vi "MasterAquisitionFile_FP_Shak.vi"() -> ()   [LabVIEW 2020]
uses:
  <vilib>/vision/driver/IMAQdx.llb/IMAQdx Camera Control Mode.ctl
  <vilib>/vision/driver/IMAQdx.llb/IMAQdx Acquisition Mode.ctl
  <vilib>/userDefined/High Color/IMAQdx.ctl
  <vilib>/vision/driver/IMAQdx.llb/IMAQdx Buffer Number Mode.ctl
  <vilib>/DAQmx/read.llb/DAQmx Read (Analog 1D Wfm NChan NSamp).vi
  <vilib>/DAQmx/create/channels.llb/DAQmx Create Channel (AI-Voltage-Basic).vi
  <vilib>/DAQmx/configure/timing.llb/DAQmx Timing (Sample Clock).vi
  <vilib>/DAQmx/configure/trigger.llb/DAQmx Start Trigger (Digital Edge).vi
  <vilib>/DAQmx/create/channels.llb/DAQmx Create Channel (CO-Pulse Generation-Frequency).vi
  <vilib>/DAQmx/configure/timing.llb/DAQmx Timing (Implicit).vi
  <vilib>/DAQmx/miscellaneous.llb/DAQmx Fill In Error Info.vi
  <vilib>/vision/driver/NI_Vision_Acquisition_Software.lvlib
  <resource>/objmgr/imaqdx.rc
panel:
  in  "Analog Input Channels":tag="Dev1/ai3:5, Dev1/ai8:13"
  out "?":T1(plugin-control)
  in  "stop":bool
  out "?":T1(plugin-control)
  out "Behavior Cam Fs":dbl(knob)=12.024443130297655 scale=0.0..200.0
  out "Behav Cam":bool=TRUE
  out "Whisk Cam":bool=TRUE
  out "Analog Data":bool=TRUE
  out "Time Elapsed (Min)":cluster{dbl, dbl}(slide)={15.0, 10.85073638} scale=0.0..16.0 scale format="%#_2g"
  out "Saving":bool
  out "Analog Samples":i32=13018238
  in  "Device Analog Channel Labels":string[](array[string])=["AudSol", "forceSensor", "560LH", "hipp", "cortRH", "cortLH", "EMG", "LPadSol", "RPadSol"]
  in  "?":cluster{"Analog Fs":u16}={"Analog Fs"=20000} {"Analog Fs" format="%0.0f"}
  in  "?":cluster{"WhiskerCam Fs":u16}={"WhiskerCam Fs"=150}
  out "Notes Size":i32=7
  out "Notes Reversed":string[](array[string])=["Experimenter", "Animal ID", "Isoflurane time", "Amplifier Gain", "Session ID", "Hemisphere", "Solenoid PSI"]
  out "Notes Array":string[](array[string])=["Solenoid PSI", "Hemisphere", "Session ID", "Amplifier Gain", "Isoflurane time", "Animal ID", "Experimenter"]
  in  "Notes:":T2={"Experimenter"="Kevin\n", "Animal ID"="T251", "Isoflurane time"="0940", "Amplifier Gain"="10000", "Session ID"="Imaging Session One", "Hemisphere"="RH", "Solenoid PSI"="10"}
  in  "Target Path":path=path "C:/LabViewData/Bilateral/T251/Imaging Session 1 - 28 Feb. 2022" caption="Final Saved File Location"
  out "Dropped":u32(slide) caption="WhiskerCam" scale=0.0..150.0
  out "Current File Name":string="220223_16_02_14"
  in  "Time (min)":dbl(knob)=15.0 min=0.5 max=20.0 step=0.5 scale=0.0..20.0 scale format="%#_3g"
  in  "Temp Path":path=path "C:/Users/mfh5734/Documents/LabVIEW Data" caption="Temporary File Path"
  out "Last Whisk Buffer":u32=97635
  out "Whisker Cam Fs":dbl(knob)=150.0 scale=0.0..200.0 scale format="%#1_6g"
  # "Notes"
  # "Dropped Frames"
  # "Analog Fs"
  # "Whisker Fs"
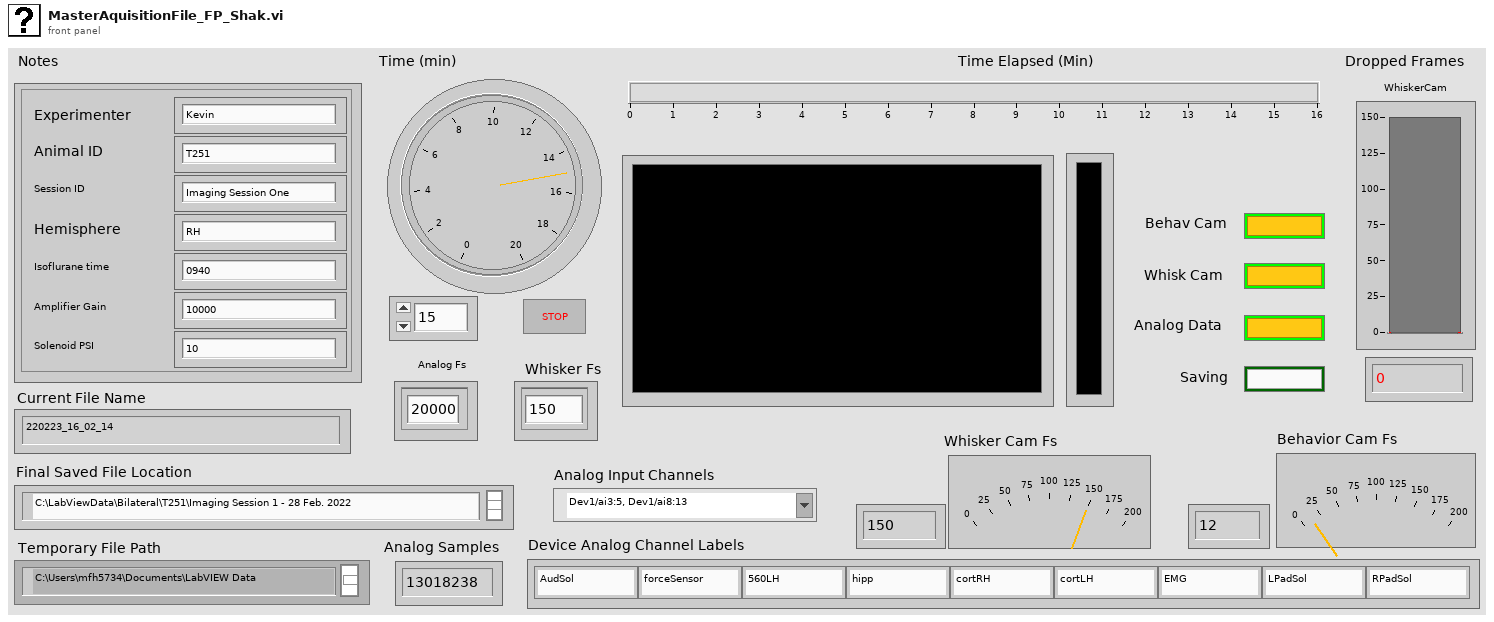
[diagram p1: front panel]
types:
  T1 = typedef "IMAQ Image.ctl" = refnum<image>
  T2 = cluster{"Experimenter":string, "Animal ID":string, "Isoflurane time":string, "Amplifier Gain":string, "Session ID":string, "Hemisphere":string, "Solenoid PSI":string}
  T3 = typedef "IMAQdx.ctl" = refnum<k21>
  T4 = enum16{"open", "open or create", "create or replace", "create", "open (read-only)"}
  T5 = typedef "NI_Vision_Acquisition_Software.lvlib/IMAQdx Camera Control Mode.ctl" = enum32{"Controller", "Listener"}
  T6 = enum16{"open", "replace", "create", "open or create", "replace or create", "replace or create with confirmation"}
  T7 = typedef "NI_Vision_Acquisition_Software.lvlib/IMAQdx Acquisition Mode.ctl" = enum32{"One Shot", "Continuous"}
  T8 = enum16{"big-endian, network order", "native, host order", "little-endian"}
  T9 = typedef "NI_Vision_Acquisition_Software.lvlib/IMAQdx Buffer Number Mode.ctl" = enum32{"Next", "Last", "Buffer Number", "Every", "Last New"}
  T10 = typedef "Image Type" = u32
  T11 = typedef "IMAQ AVI2 Refnum.ctl" = refnum<k20>
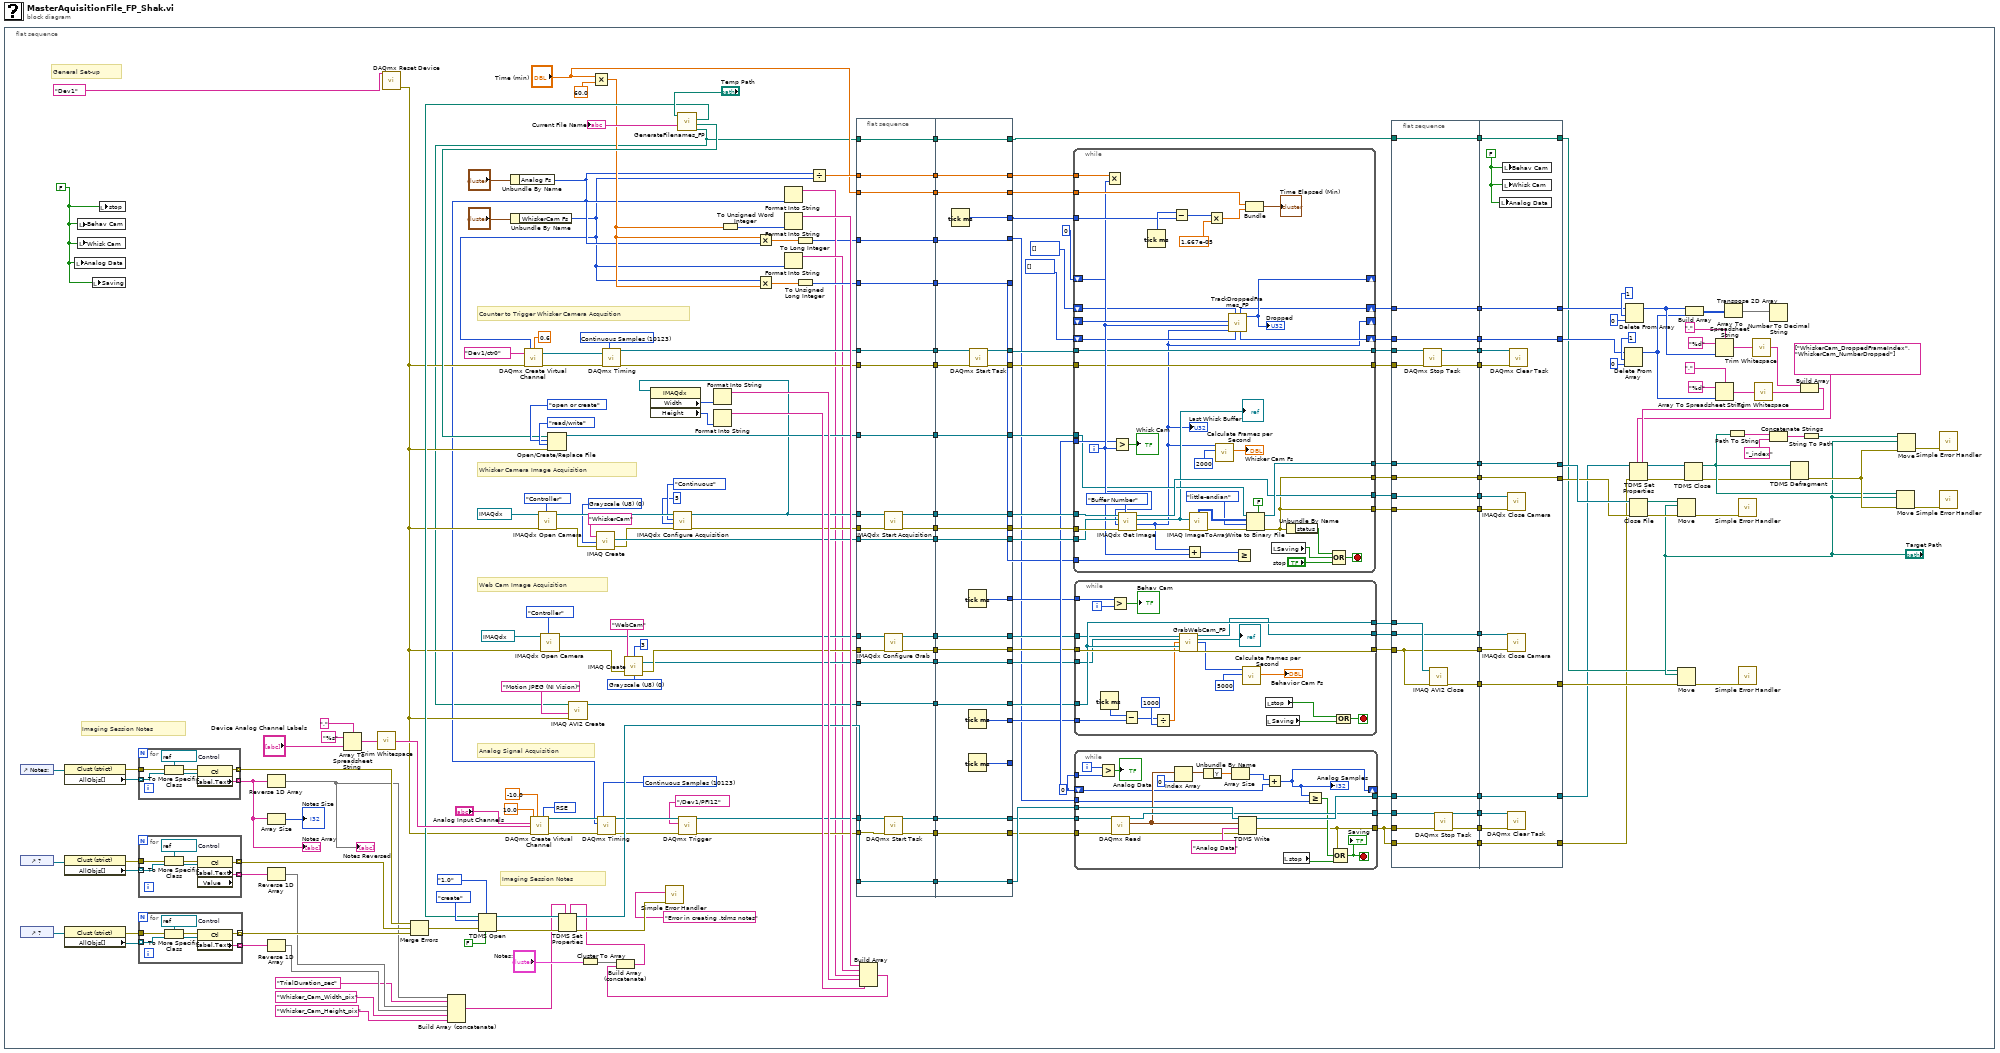
[diagram p0: block diagram]
diagram:
  n1 = flat-sequence {
    frame #0 {
      w2 = FALSE
      w117 = T10 0 items=["Grayscale (U8)", "Grayscale (I16)", "Grayscale (SGL)", "Complex (CSG)", "RGB (U32)", "HSL (U32)", "RGB (U64)", "Grayscale (U16)"] ("Image Type")
      w109 = u32 0 ("y")
      w131 = 10123 items=["Finite Samples"=10178, "Continuous Samples"=10123, "Hardware Timed Single Point"=12522] ("sample mode")
      w130 = 10083 items=["default"=-1, "RSE"=10083, "NRSE"=10078, "Differential"=10106, "Pseudodifferential"=12529] ("input terminal configuration")
      w132 = 10123 items=["Finite Samples"=10178, "Continuous Samples"=10123, "Hardware Timed Single Point"=12522] ("sample mode")
      w128 = T10 0 items=["Grayscale (U8)", "Grayscale (I16)", "Grayscale (SGL)", "Complex (CSG)", "RGB (U32)", "HSL (U32)", "RGB (U64)", "Grayscale (U16)"] ("Image Type")
      # "General Set-up"
      # "Imaging Session Notes"
      # "Whisker Camera Image Acquisition"
      # "Imaging Session Notes"
      # "Counter to Trigger Whisker Camera Acqusition"
      # "Web Cam Image Acquisition"
      # "Analog Signal Acquisition"
      n2 = control-ref of="Notes:"() -> (w69:refnum<vi>)
      n3 = control-ref of="?"() -> (w71:refnum<vi>)
      n4 = control-ref of="?"() -> (w78:refnum<vi>)
      n5 = property class="Clust (strict)"(reference=w69) -> (error out=w70:errorcluster, "AllObjs[]"=w68:refnum<vi>[])  [unwired: 1 in, 1 out]
      n6 = property class="Clust (strict)"(reference=w71) -> (error out=w73:errorcluster, "AllObjs[]"=w72:refnum<vi>[])  [unwired: 1 in, 1 out]
      n7 = property class="Clust (strict)"(reference=w78) -> (error out=w77:errorcluster, "AllObjs[]"=w75:refnum<vi>[])  [unwired: 1 in, 1 out]
      n8 = local write "Analog Data"(w2) -> ()
      n9 = local write "Behav Cam"(w2) -> ()
      n10 = local write "Whisk Cam"(w2) -> ()
      n11 = local write "Saving"(w2) -> ()
      n12 = local write "stop"(w2) -> ()
      n13 = for {
        tunnel: [w234] -> w63 mode=indexing
        tunnel: w68 -> [w233] mode=indexing
        tunnel: w70 -> [w232]
        tunnel: [w230] -> w64 mode=indexing
        w235 = refnum<vi> refnum  # Control
        n14 = To More Specific Class(target class=w235, reference=w233, error in=w232) -> (specific class reference=w236:refnum<vi>, error out=w231:errorcluster)
        n15 = property class="Ctl"(reference=w236, error in=w231) -> (error out=w230:errorcluster, "Label.Text"=w234:string)  [unwired: 1 out]
      }
      "Notes Array" <- w63
      n16 = for {
        tunnel: [w241] -> w74 mode=indexing
        tunnel: w72 -> [w240] mode=indexing
        tunnel: w73 -> [w239]
        tunnel: [w237] -> w65 mode=indexing
        w242 = refnum<vi> refnum  # Control
        n17 = To More Specific Class(target class=w242, reference=w240, error in=w239) -> (specific class reference=w243:refnum<vi>, error out=w238:errorcluster)
        n18 = property class="Ctl" props=["Label", "Text", "Value"](reference=w243, error in=w238) -> (error out=w237:errorcluster, "Label.Text"=w241:string)  [unwired: 2 out]
      }
      n19 = for {
        tunnel: [w248] -> w76 mode=indexing
        tunnel: w75 -> [w247] mode=indexing
        tunnel: w77 -> [w246]
        tunnel: [w244] -> w66 mode=indexing
        w249 = refnum<vi> refnum  # Control
        n20 = To More Specific Class(target class=w249, reference=w247, error in=w246) -> (specific class reference=w250:refnum<vi>, error out=w245:errorcluster)
        n21 = property class="Ctl"(reference=w250, error in=w245) -> (error out=w244:errorcluster, "Label.Text"=w248:string)  [unwired: 1 out]
      }
      n22 = Reverse 1D Array(array=w63) -> (reversed array=w62:string[])
      "Notes Reversed" <- w62
      n23 = Array Size(array=w63) -> (size(s)=→"Notes Size":i32)
      n24 = Reverse 1D Array(array=w74) -> (reversed array=w58:string[])
      n25 = Reverse 1D Array(array=w76) -> (reversed array=w57:string[])
      n26 = Array To Spreadsheet String(delimiter (Tab)=",", array="Device Analog Channel Labels", 3:"%s" ("format string")) -> (spreadsheet string=w61:string)
      n27 = call <vilib>:"Trim Whitespace.vi"("string"=w61) -> ("trimmed string"=w50:string)  [unwired: 1 in]
      n28 = call <vilib>:"DAQmx Reset Device.vi"("device in"=tag "Dev1" ("NI Board")) -> ("error out"=w33:errorcluster)  [unwired: 14 in]
      n29 = Merge Errors(w64, w65, w66) -> (w49:errorcluster)
      n30 = Build Array (concatenate)(w62, "TrialDuration_sec", w58, w57, "Whisker_Cam_Width_pix", "Whisker_Cam_Height_pix") -> (w48:string[])
      n31 = Unbundle By Name("?") -> ("Analog Fs"=w31:u16)
      n32 = Unbundle By Name("?") -> ("WhiskerCam Fs"=w30:u16)
      n33 = call-poly <vilib>:"DAQmx Create Virtual Channel.vi"("frequency"=w30, "duty cycle"=0.6, "counter"=tag "Dev1/ctr0" ("Whisk Cam Counter"), "error in"=w33) -> ("task out"=w155:refnum<k21>, "error out"=w156:errorcluster)  [unwired: 10 in]
      n34 = call-poly <vilib>:"DAQmx Create Virtual Channel.vi"("maximum value"=10.0, "minimum value"=-10.0, "input terminal configuration"=w130, "physical channels"="Analog Input Channels", "name to assign"=w50, "error in"=w33) -> ("task out"=w163:refnum<k21>, "error out"=w164:errorcluster)  [unwired: 8 in]
      n35 = call <vilib>:"IMAQdx Open Camera.vi"("Camera Control Mode"=IMAQdx_Camera_Control_Mode."Controller", "error in"=w33, "Session In"=T3 "cam1" ("Whisker Cam ID")) -> ("error out"=w153:errorcluster, "Session Out"=w152:T3)  [unwired: 7 in]
      n36 = call <vilib>:"IMAQdx Open Camera.vi"("Camera Control Mode"=IMAQdx_Camera_Control_Mode."Controller", "error in"=w33, "Session In"=T3 "cam2" ("WebCam ID")) -> ("error out"=w114:errorcluster, "Session Out"=w113:T3)  [unwired: 7 in]
      n37 = Cluster To Array(cluster="Notes:") -> (array=w51:string[])
      n38 = Multiply(x="Time (min)", y=60.0) -> (x*y=w32:dbl)
      n39 = call "IMAQ Create"("Image Name"="WhiskerCam", "Image Type"=w128, "error in (no error)"=w153) -> ("New Image"=w188:T1, "error out"=w154:errorcluster)  [unwired: 2 in]
      n40 = call-poly <vilib>:"DAQmx Timing.vi"("task/channels in"=w163, "sample mode"=w131, "rate"=w31, "error in"=w164) -> ("task out"=w165:refnum<k21>, "error out"=w166:errorcluster)  [unwired: 10 in]
      n41 = call-poly <vilib>:"DAQmx Timing.vi"("task/channels in"=w155, "sample mode"=w132, "error in"=w156) -> ("task out"=w172:refnum<k21>, "error out"=w173:errorcluster)  [unwired: 11 in]
      n42 = call "IMAQ Create"("Border Size"=3, "Image Name"="WebCam", "Image Type"=w117, "error in (no error)"=w114) -> ("New Image"=w111:T1, "error out"=w112:errorcluster)  [unwired: 1 in]
      n43 = call <vilib>:"IMAQdx Configure Acquisition.vi"("error in"=w154, "Number of Buffers"=u32 5, "Continuous?"=IMAQdx_Acquisition_Mode."Continuous", "Session In"=w152) -> ("error out"=w157:errorcluster, "Session Out"=w97:T3)  [unwired: 6 in]
      n44 = property class="IMAQdx"(reference=w97) -> ("Width"=w186:u32, "Height"=w187:u32)  [unwired: 1 in, 2 out]
      n45 = call "GenerateFilenames_FP.vi"("path"="Temp Path") -> ("WebCam Path"=w13:path, "Basler Path"=w38:path, "TDMS Path"=w37:path, "Analog file name"=→"Current File Name":string)  [unwired: 2 in, 1 out]
      n46 = TDMS Open(6:FALSE ("disable buffering? (T)"), 7:enum16{"1.0", "2.0"}."1.0" ("file format version (2.0)"), 8:w49, 10:T4."create" ("operation (0:open)"), 11:w37) -> (0:w99:errorcluster, 3:w98:refnum<k34>)  [unwired: 2 in]
      n47 = Open/Create/Replace File(file path (use dialog)=w38, error in=w33, operation (0:open)=T6."open or create", access (0:read/write)=enum16{"read/write", "read-only", "write-only"}."read/write") -> (refnum out=w162:refnum<file>)  [unwired: 2 in, 2 out]
      n48 = call "IMAQ AVI2 Create"("error in (no error)"=w33, "Codec"="Motion JPEG (NI Vision)", "AVI Path"=w13) -> ("AVI Refnum"=w105:T11)  [unwired: 7 in, 1 out]
      n49 = call-poly <vilib>:"DAQmx Trigger.vi"("task/channels in"=w165, "source"=tag "/Dev1/PFI12" ("Whisk Cam Trigger"), "error in"=w166) -> ("task out"=w167:refnum<k21>, "error out"=w168:errorcluster)  [unwired: 11 in]
      n50 = Format Into String(w186) -> (resulting string=w202:string)  [unwired: 3 in, 1 out]
      n51 = Format Into String(w187) -> (resulting string=w201:string)  [unwired: 3 in, 1 out]
      n52 = To Unsigned Word Integer(number=w32) -> (unsigned 16bit integer=w185:u16)
      n53 = Multiply(x=w32, y=w31) -> (x*y=w15:dbl)
      n54 = Multiply(x=w30, y=w32) -> (x*y=w195:dbl)
      n55 = Format Into String(w31) -> (resulting string=w34:string)  [unwired: 3 in, 1 out]
      n56 = Format Into String(w185) -> (resulting string=w203:string)  [unwired: 3 in, 1 out]
      n57 = Format Into String(w30) -> (resulting string=w35:string)  [unwired: 3 in, 1 out]
      n58 = To Long Integer(number=w15) -> (32bit integer=w14:i32)
      n59 = To Unsigned Long Integer(number=w195) -> (unsigned 32bit integer=w196:u32)
      n60 = Divide ("An_Fs/Whisk_Fs ratio")(x=w31, y=w30) -> (x/y=w39:dbl)
      n61 = flat-sequence {
        tunnel: w97 -> [w355]
        tunnel: w157 -> [w354]
        tunnel: [w353] -> w229
        tunnel: [w352] -> w228
        tunnel: [w351] -> w227
        tunnel: w188 -> [w351]
        tunnel: [w350] -> w226
        tunnel: w162 -> [w350]
        tunnel: w167 -> [w349]
        tunnel: w168 -> [w348]
        tunnel: [w347] -> w225
        tunnel: [w346] -> w224
        tunnel: [w345] -> w223
        tunnel: w183 -> [w345]
        tunnel: w172 -> [w344]
        tunnel: [w344] -> w222
        tunnel: w173 -> [w343]
        tunnel: [w343] -> w221
        tunnel: w14 -> [w342]
        tunnel: [w342] -> w220
        tunnel: w196 -> [w341]
        tunnel: [w341] -> w219
        tunnel: "Time (min)" -> [w340]
        tunnel: [w340] -> w218
        tunnel: w113 -> [w339]
        tunnel: w112 -> [w338]
        tunnel: w111 -> [w337]
        tunnel: [w337] -> w217
        tunnel: [w336] -> w216
        tunnel: [w335] -> w215
        tunnel: [w334] -> w214
        tunnel: w105 -> [w334]
        tunnel: [w333] -> w213
        tunnel: w39 -> [w333]
        tunnel: w13 -> [w332]
        tunnel: [w332] -> w12
        tunnel: [w372] -> w121
        tunnel: [w371] -> w122
        tunnel: [w379] -> w158
        tunnel: w229 -> [w379]
        tunnel: [w378] -> w159
        tunnel: w228 -> [w378]
        tunnel: [w377] -> w160
        tunnel: w227 -> [w377]
        tunnel: [w376] -> w161
        tunnel: w226 -> [w376]
        tunnel: [w375] -> w170
        tunnel: w225 -> [w375]
        tunnel: [w374] -> w169
        tunnel: w224 -> [w374]
        tunnel: [w373] -> w171
        tunnel: w223 -> [w373]
        tunnel: w222 -> [w368]
        tunnel: w221 -> [w370]
        tunnel: w220 -> [w357]
        tunnel: w219 -> [w369]
        tunnel: [w369] -> w94
        tunnel: [w367] -> w151
        tunnel: w218 -> [w366]
        tunnel: [w366] -> w120
        tunnel: [w365] -> w108
        tunnel: w217 -> [w365]
        tunnel: [w364] -> w106
        tunnel: w216 -> [w364]
        tunnel: [w363] -> w107
        tunnel: w215 -> [w363]
        tunnel: [w362] -> w103
        tunnel: w214 -> [w361]
        tunnel: [w361] -> w104
        tunnel: [w360] -> w102
        tunnel: [w357] -> w93
        tunnel: [w359] -> _
        tunnel: [w358] -> w88
        tunnel: w213 -> [w358]
        tunnel: [w356] -> w10
        tunnel: w12 -> [w356]
        frame #0 {
          n62 = call <vilib>:"IMAQdx Start Acquisition.vi"("error in"=w354, "Session In"=w355) -> ("error out"=w352:errorcluster, "Session Out"=w353:T3)  [unwired: 8 in]
          n63 = call <vilib>:"IMAQdx Configure Grab.vi"("error in"=w338, "Session In"=w339) -> ("error out"=w335:errorcluster, "Session Out"=w336:T3)  [unwired: 8 in]
          n64 = call <vilib>:"DAQmx Start Task.vi"("task/channels in"=w349, "error in"=w348) -> ("task out"=w347:refnum<k21>, "error out"=w346:errorcluster)  [unwired: 12 in]
        }
        frame #1 {
          n65 = Tick Count (ms)() -> (millisecond timer value=w367:u32)
          n66 = Tick Count (ms)() -> (millisecond timer value=w362:u32)
          n67 = Tick Count (ms)() -> (millisecond timer value=w360:u32)
          n68 = Tick Count (ms)() -> (millisecond timer value=w359:u32)
          n69 = call <vilib>:"DAQmx Start Task.vi"("task/channels in"=w368, "error in"=w370) -> ("task out"=w372:refnum<k21>, "error out"=w371:errorcluster)  [unwired: 12 in]
        }
      }
      n70 = Build Array(w203, w35, w34, w202, w201) -> (w95:string[])
      n71 = Build Array (concatenate)(w51, w95) -> (w123:string[])
      n72 = TDMS Set Properties(5:w123, 7:w48, 8:w99, 11:w98) -> (0:w184:errorcluster, 3:w183:refnum<k34>)  [unwired: 2 in, 2 out]
      n73 = call <vilib>:"Simple Error Handler.vi"("error source (\" \")"="Error in creating .tdms notes" ("error source (\" \")"), "error in (no error)"=w184) -> ()  [unwired: 3 in, 5 out]
      n74 = while {
        tunnel: [w407] -> w79
        tunnel: [w393] -> w17
        tunnel: [w415] -> w20
        tunnel: w158 -> [w414]
        tunnel: w159 -> [w413]
        tunnel: w160 -> [w412]
        tunnel: w161 -> [w387]
        shift-right: [w384] -> _
        shift-left: _ -> [w411]
        shift-right: [w410] -> _
        shift-left: u32 0 ("New Lost") -> [w406]
        shift-right: [w409] -> w26
        shift-left: u32[] [] ("NewBuffNum") -> [w383]
        shift-right: [w408] -> w22
        shift-left: u32[] [] ("NewNumLost") -> [w402]
        tunnel: w94 -> [w404]
        tunnel: w151 -> [w397]
        tunnel: w120 -> [w395]
        tunnel: [w393] -> w80
        tunnel: w109 -> [w392]
        tunnel: w122 -> [w390]
        tunnel: w121 -> [w389]
        tunnel: [w390] -> w86
        tunnel: [w389] -> w87
        tunnel: w88 -> [w385]
        i -> [w382]
        stop <- w403 stop-if-true
        n75 = Multiply(x=w385, y=w382) -> ()  [unwired: 1 out]
        n76 = Greater?(x=w382, y=w392) -> (0:→"Whisk Cam":bool)
        n77 = call <vilib>:"IMAQdx Get Image.vi"("Buffer Number Mode (Next)"=IMAQdx_Buffer_Number_Mode."Buffer Number", "error in"=w413, "Buffer Number In"=w382, "Image In"=w412, "Session In"=w414) -> ("error out"=w421:errorcluster, "Buffer Number Out"=w384:u32, "Image Out"=w386:T1, "Session Out"=w407:T3)  [unwired: 3 in]
        "Last Whisk Buffer" <- w384
        "?" <- w386
        n78 = Tick Count (ms)() -> (millisecond timer value=w398:u32)
        n79 = Subtract(x=w398, y=w397) -> (x-y=w401:u32)
        n80 = Add(x=w384, y=w406) -> (x+y=w405:u32)
        n81 = call "IMAQ ImageToArray"("error in (no error)"=w421, "Image"=w386) -> ("error out"=w420:errorcluster, "Image Pixels (U8)"=w419:u8[][])  [unwired: 2 in, 3 out]
        n82 = Multiply(x=w401, y=1.667e-05) -> (x*y=w400:dbl)
        n83 = call <vilib>:"Calculate Frames per Second.vi"("Update Interval (ms)"=u32 2000, "Buffer Number"=w384) -> ("Processed Frames/s"=→"Whisker Cam Fs":dbl)  [unwired: 7 in, 2 out]
        n84 = call "TrackDroppedFrames_FP.vi"("NumLost"=w402, "BuffNum"=w383, "Curr Buffer"=w384, "Prev Lost"=w406, "Prev Buffer"=w411) -> ("New Lost"=w410:u32, "NewNumLost"=w408:u32[], "NewBuffNum"=w409:u32[])  [unwired: 4 in]
        "Dropped" <- w410
        n85 = Greater Or Equal?(x=w405, y=w404) -> ()  [unwired: 1 out]
        n86 = Bundle("Time (min)"=w395, w400) -> (→"Time Elapsed (Min)":cluster{"Time (min)":dbl, dbl})  [unwired: 1 in]
        n87 = Write to Binary File(file (use dialog)=w387, data=w419, error in=w420, 5:FALSE ("prepend array or string size? (T)"), 9:T8."little-endian" ("byte order (0:big-endian, network order)")) -> (refnum out=w415:refnum<file>, error out=w393:errorcluster)  [unwired: 1 in, 1 out]
        n88 = local read "Saving"() -> (w380:bool)
        n89 = Unbundle By Name(w393) -> ("status"=w381:bool)
        n90 = Compound Arithmetic op=OR(w381, w380, "stop") -> (w403:bool)
      }
      n91 = while {
        tunnel: w169 -> [w331]
        tunnel: w170 -> [w330]
        tunnel: w171 -> [w329]
        tunnel: [w328] -> w7
        tunnel: [w316] -> w5
        tunnel: [w327] -> w85
        shift-right: [w320] -> _
        shift-left: w109 -> [w321]
        tunnel: w109 -> [w312]
        tunnel: w93 -> [w310]
        i -> [w313]
        stop <- w317 stop-if-true
        n92 = Greater?(x=w313, y=w312) -> (0:→"Analog Data":bool)
        n93 = call-poly <vilib>:"DAQmx Read.vi"("task/channels in"=w330, "error in"=w331) -> ("task out"=w327:refnum<k21>, "data"=w325:waveform(dbl)[], "error out"=w319:errorcluster)  [unwired: 11 in]
        n94 = Index Array(array=w325, index=0) -> (element=w323:waveform(dbl))
        n95 = Unbundle By Name(w323) -> ("Y"=w322:dbl[])
        n96 = Array Size(array=w322) -> (size(s)=w315:i32)
        n97 = TDMS Write(0:w329, 5:"Analog Data" ("group name in (Untitled)"), 9:w325, 11:w319) -> (4:w328:refnum<k34>, 15:w316:errorcluster)  [unwired: 2 in, 2 out]
        n98 = Add(x=w315, y=w321) -> (x+y=w320:u32)
        "Analog Samples" <- w320
        n99 = local read "stop"() -> (w311:bool)
        n100 = Greater Or Equal?(x=w320, y=w310) -> (x >= y?=w318:bool)
        n101 = Compound Arithmetic op=OR(w311, w316, w318) -> (w317:bool)
        "Saving" <- w317
      }
      n102 = while {
        tunnel: w108 -> [w296]
        tunnel: w106 -> [w295]
        tunnel: w107 -> [w299]
        tunnel: w104 -> [w298]
        tunnel: [w289] -> w81
        tunnel: [w300] -> w82
        tunnel: [w298] -> w84
        tunnel: w103 -> [w302]
        tunnel: w102 -> [w301]
        i -> [w303]
        stop <- w291 stop-if-true
        n103 = Tick Count (ms)() -> (millisecond timer value=w307:u32)
        n104 = Greater?(x=w302, y=w303) -> (0:→"Behav Cam":bool)
        n105 = Subtract(x=w307, y=w301) -> (x-y=w308:u32)
        n106 = Divide(x=w308, y=u32 1000) -> (x/y=w297:dbl)
        n107 = call "GrabWebCam_FP.vi"("Session In"=w295, "Image In"=w296, "Trial Time"=w297, "AVI Refnum"=w298, "error in"=w299) -> ("Session Out"=w289:T3, "WebCam Img Out"=→"?":T1, "Buffer Number Out"=w293:u32, "error out"=w300:errorcluster)  [unwired: 7 in]
        n108 = call <vilib>:"Calculate Frames per Second.vi"("Update Interval (ms)"=u32 5000, "Buffer Number"=w293) -> ("Processed Frames/s"=→"Behavior Cam Fs":dbl)  [unwired: 7 in, 2 out]
        n109 = local read "stop"() -> (w290:bool)
        n110 = local read "Saving"() -> (w292:bool)
        n111 = Compound Arithmetic op=OR(w290, w292) -> (w291:bool)
      }
      n112 = flat-sequence {
        tunnel: w87 -> [w271]
        tunnel: w86 -> [w270]
        tunnel: [w269] -> w212
        tunnel: [w268] -> w211
        tunnel: [w267] -> w210
        tunnel: [w266] -> w209
        tunnel: w85 -> [w265]
        tunnel: w5 -> [w264]
        tunnel: w82 -> [w260]
        tunnel: w84 -> [w263]
        tunnel: [w262] -> w208
        tunnel: [w261] -> w207
        tunnel: w81 -> [w261]
        tunnel: [w260] -> w206
        tunnel: w80 -> [w259]
        tunnel: [w259] -> w205
        tunnel: w79 -> [w258]
        tunnel: [w258] -> w204
        tunnel: w26 -> [w257]
        tunnel: [w257] -> w25
        tunnel: [w256] -> w23
        tunnel: w22 -> [w256]
        tunnel: [w255] -> w21
        tunnel: w20 -> [w255]
        tunnel: [w254] -> w18
        tunnel: w17 -> [w254]
        tunnel: [w253] -> w11
        tunnel: w10 -> [w253]
        tunnel: w7 -> [w252]
        tunnel: [w252] -> w6
        tunnel: w5 -> [w251]
        tunnel: [w251] -> w4
        tunnel: w212 -> [w288]
        tunnel: w211 -> [w287]
        tunnel: w210 -> [w286]
        tunnel: w209 -> [w285]
        tunnel: w208 -> [w284]
        tunnel: [w284] -> w83
        tunnel: w207 -> [w283]
        tunnel: w206 -> [w282]
        tunnel: w205 -> [w281]
        tunnel: w204 -> [w280]
        tunnel: [w278] -> w27
        tunnel: w25 -> [w278]
        tunnel: [w277] -> w24
        tunnel: w23 -> [w277]
        tunnel: [w276] -> w19
        tunnel: w21 -> [w276]
        tunnel: w18 -> [w275]
        tunnel: [w275] -> w16
        tunnel: w11 -> [w274]
        tunnel: [w274] -> w9
        tunnel: [w273] -> w8
        tunnel: w6 -> [w273]
        tunnel: [w272] -> w3
        tunnel: w4 -> [w272]
        frame #0 {
          n113 = call <vilib>:"DAQmx Stop Task.vi"("task/channels in"=w271, "error in"=w270) -> ("task out"=w268:refnum<k21>, "error out"=w269:errorcluster)  [unwired: 12 in]
          n114 = call "IMAQ AVI2 Close"("error in (no error)"=w260, "AVI Refnum"=w263) -> ("error out"=w262:errorcluster)  [unwired: 9 in]
          n115 = call <vilib>:"DAQmx Stop Task.vi"("task/channels in"=w265, "error in"=w264) -> ("task out"=w267:refnum<k21>, "error out"=w266:errorcluster)  [unwired: 12 in]
        }
        frame #1 {
          w279 = FALSE
          n116 = local write "Analog Data"(w279) -> ()
          n117 = local write "Behav Cam"(w279) -> ()
          n118 = local write "Whisk Cam"(w279) -> ()
          n119 = call <vilib>:"IMAQdx Close Camera.vi"("error in"=w281, "Session In"=w280) -> ()  [unwired: 9 in, 1 out]
          n120 = call <vilib>:"IMAQdx Close Camera.vi"("error in"=w282, "Session In"=w283) -> ()  [unwired: 9 in, 1 out]
          n121 = call <vilib>:"DAQmx Clear Task.vi"("task in"=w286, "error in"=w285) -> ()  [unwired: 13 in, 1 out]
          n122 = call <vilib>:"DAQmx Clear Task.vi"("task in"=w287, "error in"=w288) -> ()  [unwired: 13 in, 1 out]
        }
      }
      n123 = Delete From Array(array=w24, length=1, index=0) -> (array with subset deleted=w199:u32[])  [unwired: 1 out]
      n124 = Delete From Array(array=w27, length=1, index=0) -> (array with subset deleted=w200:u32[])  [unwired: 1 out]
      n125 = Close File(refnum=w19, error in=w16) -> (path=w175:path, error out=w176:errorcluster)
      n126 = Move(source path=w175, error in=w176, 10:"Target Path") -> (error out=w178:errorcluster)  [unwired: 2 in, 2 out]
      n127 = Move(source path=w9, error in=w83, 10:"Target Path") -> (error out=w110:errorcluster)  [unwired: 2 in, 2 out]
      n128 = Build Array(w200, w199) -> (w197:u32[][])
      n129 = Array To Spreadsheet String(delimiter (Tab)=",", array=w200, 3:"%d" ("format string")) -> (spreadsheet string=w191:string)
      n130 = Array To Spreadsheet String(delimiter (Tab)=",", array=w199, 3:"%d" ("format string")) -> (spreadsheet string=w192:string)
      n131 = Transpose 2D Array(2D array=w197) -> (transposed array=w198:u32[][])
      n132 = call <vilib>:"Simple Error Handler.vi"("error in (no error)"=w178) -> ()  [unwired: 1 in, 8 out]
      n133 = call <vilib>:"Simple Error Handler.vi"("error in (no error)"=w110) -> ()  [unwired: 1 in, 8 out]
      n134 = call <vilib>:"Trim Whitespace.vi"("string"=w191) -> ("trimmed string"=w92:string)  [unwired: 1 in]
      n135 = call <vilib>:"Trim Whitespace.vi"("string"=w192) -> ("trimmed string"=w193:string)  [unwired: 1 in]
      n136 = Number To Decimal String(number=w198) -> ()  [unwired: 1 in, 1 out]
      n137 = Build Array(w92, w193) -> (w194:string[])
      n138 = TDMS Set Properties(5:w194, 7:string[] ["WhiskerCam_DroppedFrameIndex", "WhiskerCam_NumberDropped"] ("channel name(s) in (Untitled)"), 8:w3, 11:w8) -> (0:w189:errorcluster, 3:w190:refnum<k34>)  [unwired: 2 in, 2 out]
      n139 = TDMS Close(8:w189, 11:w190) -> (0:w174:errorcluster, 3:w179:path)
      n140 = Path To String(path=w179) -> (string=w91:string)
      n141 = Concatenate Strings(w91, "_index" ("string")) -> (w180:string)
      n142 = TDMS Defragment(4:w174, 7:w179) -> (0:w182:errorcluster)
      n143 = String To Path(string=w180) -> (path=w181:path)
      n144 = Move(source path=w179, error in=w182, 10:"Target Path") -> (error out=w177:errorcluster)  [unwired: 2 in, 2 out]
      n145 = Move(source path=w181, error in=w182, 10:"Target Path") -> (error out=w90:errorcluster)  [unwired: 2 in, 2 out]
      n146 = call <vilib>:"Simple Error Handler.vi"("error in (no error)"=w90) -> ()  [unwired: 1 in, 8 out]
      n147 = call <vilib>:"Simple Error Handler.vi"("error in (no error)"=w177) -> ()  [unwired: 1 in, 8 out]
    }
  }
